vi "Autoignition McKay.vi"() -> ()   [LabVIEW 2014]
uses:
  <vilib>/Analysis/baseanly.llb/Mean (DBL).vi
  <vilib>/Utility/file.llb/Write To Spreadsheet File (DBL).vi
  <vilib>/Analysis/NI_AALBase.lvlib
panel:
  out "Data Collection":bool
  in  "file path (dialog if empty)":path=path "c:/temp/trial1"
  in  "?":bool
  out "Waveform Chart":dynamicdata(graph)
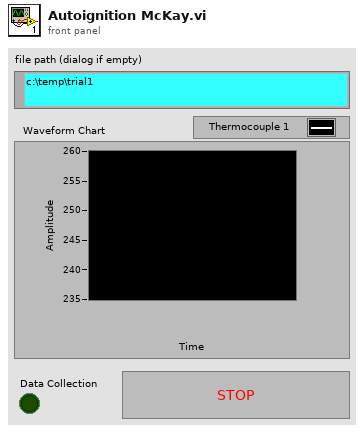
[diagram p1: front panel]
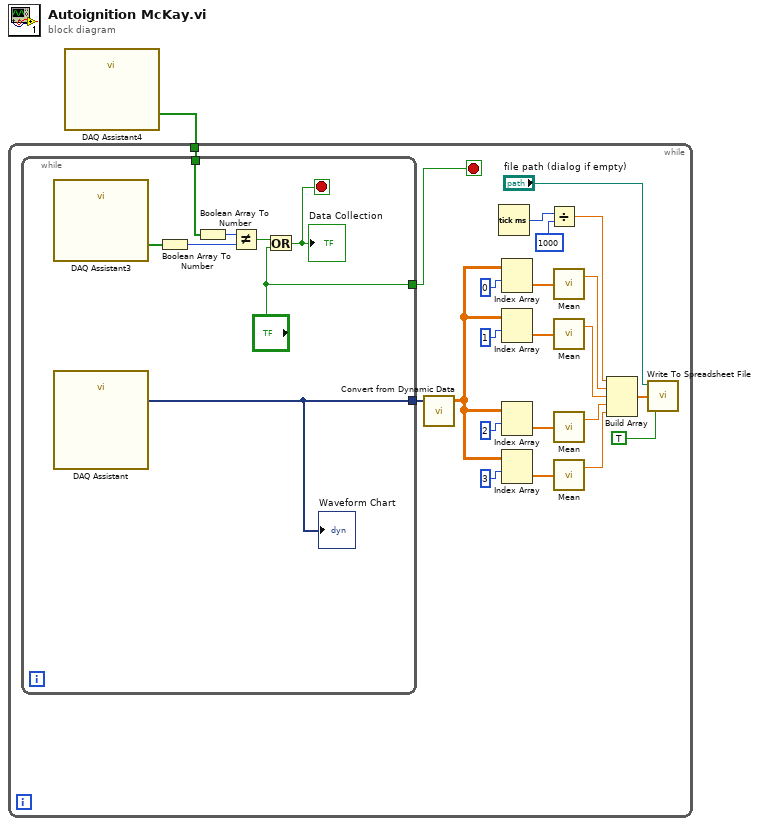
[diagram p0: block diagram]
diagram:
  n1 = call "DAQ Assistant4"() -> ("data"=w1:bool[])  [unwired: 17 in, 2 out]
  n2 = while {
    tunnel: w1 -> [w13]
    stop <- w12 stop-if-true
    n3 = while {
      tunnel: ["?"] -> w12
      tunnel: [w31] -> w3
      tunnel: w13 -> [w28]
      stop <- w29 stop-if-true
      n4 = call "DAQ Assistant3"() -> ("data"=w25:bool[])  [unwired: 17 in, 2 out]
      n5 = call "DAQ Assistant"() -> ("data"=w31:dynamicdata)  [unwired: 17 in, 2 out]
      "Waveform Chart" <- w31
      n6 = Boolean Array To Number(Boolean array=w25) -> (number=w27:u32)
      n7 = Boolean Array To Number(Boolean array=w28) -> (number=w26:u32)
      n8 = Not Equal?(x=w26, y=w27) -> (x != y?=w24:bool)
      n9 = Or(x=w24, y="?") -> (x .or. y?=w29:bool)
      "Data Collection" <- w29
    }
    n10 = call "Convert from Dynamic Data"("Dynamic Data Type"=w3) -> ("Array"=w2:dbl[][])  [unwired: 3 in]
    n11 = Tick Count (ms)() -> (millisecond timer value=w16:u32)
    n12 = Index Array(array=w2, index (row)=0) -> (element=w18:dbl[])  [unwired: 1 in]
    n13 = Index Array(array=w2, index (row)=1) -> (element=w19:dbl[])  [unwired: 1 in]
    n14 = Index Array(array=w2, index (row)=2) -> (element=w20:dbl[])  [unwired: 1 in]
    n15 = Index Array(array=w2, index (row)=3) -> (element=w21:dbl[])  [unwired: 1 in]
    n16 = Divide(x=w16, y=1000) -> (x/y=w14:dbl)
    n17 = call-poly <vilib>:"Mean.vi"("X"=w18) -> ("mean"=w7:dbl)  [unwired: 1 out]
    n18 = call-poly <vilib>:"Mean.vi"("X"=w19) -> ("mean"=w6:dbl)  [unwired: 1 out]
    n19 = call-poly <vilib>:"Mean.vi"("X"=w20) -> ("mean"=w5:dbl)  [unwired: 1 out]
    n20 = call-poly <vilib>:"Mean.vi"("X"=w21) -> ("mean"=w4:dbl)  [unwired: 1 out]
    n21 = Build Array(w14, w7, w6, w5, w4) -> (w22:dbl[])
    n22 = call-poly <vilib>:"Write To Spreadsheet File.vi"("append to file? (new file:F)"=TRUE, "1D data"=w22, "file path (dialog if empty)"="file path (dialog if empty)") -> ()  [unwired: 5 in, 1 out]
  }
